vi "Construct Boolean Text Binding.vi"(7 "Format String":string, 10 "Bool Refnum":refnum<vi>) -> (0 "error out":errorcluster, 3 "BooleanTextBinding":refnum<class "BooleanTextBinding.lvclass">)   [LabVIEW 2020, in "BooleanTextBinding.lvclass"]
doc: "构造布尔文本绑定"
uses:
  BooleanTextBinding.lvclass
  BooleanTextBinding.lvclass/BooleanTextBinding.ctl
  <vilib>/Utility/error.llb/Error Cluster From Error Code.vi
  <vilib>/ErrorRing/Error Ring.xnode
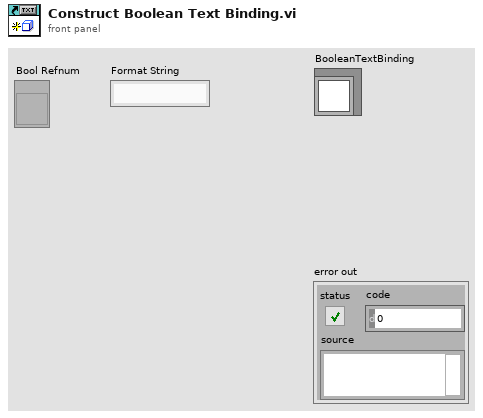
[diagram p1: front panel]
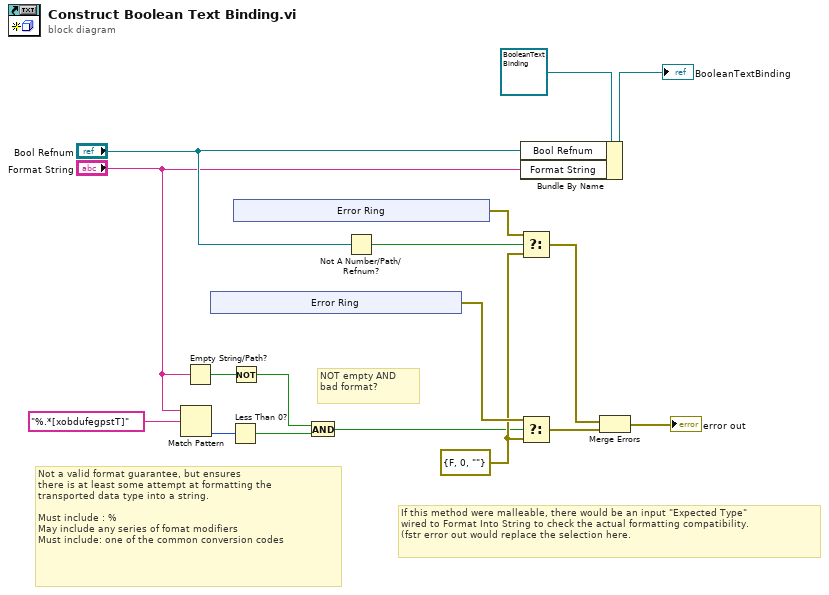
[diagram p0: block diagram]
diagram:
  w6 = errorcluster {"status"=FALSE, "code"=0, "source"=""} ("error constant")
  # "NOT empty AND\nbad format?"
  # "If this method were malleable, there would be an input \"Expected Type\"\nwired to Format Into String to check the actual formatting compatibility.\n(fstr error out would replace the selection here."
  # "Not a valid format guarantee, but ensures\nthere is at least some attempt at formatting the\ntransported data type into a string.\n\nMust include : %\nMay include any series of fomat modifiers\nMust include: one of the common conversion codes"
  n1 = Match Pattern(string="Format String", regular expression="%.*[xobdufegpstT]") -> (offset past match=w11:i32)  [unwired: 1 in, 3 out]
  n2 = Empty String/Path?(string/path="Format String") -> (empty?=w5:bool)
  n3 = xnode "Error Ring"() -> ("error out"=w10:errorcluster)
  n4 = Less Than 0?(x=w11) -> (x < 0?=w2:bool)
  n5 = Not(x=w5) -> (.not. x?=w4:bool)
  n6 = xnode "Error Ring"() -> ("error out"=w15:errorcluster)
  n7 = And(x=w4, y=w2) -> (x .and. y?=w1:bool)
  n8 = Not A Number/Path/Refnum?(number/path/refnum="Bool Refnum") -> (NaN/Path/Refnum?=w13:bool)
  n9 = Bundle By Name(cluster=refnum<class "BooleanTextBinding.lvclass"> refnum ("BooleanTextBinding"), "Bool Refnum"="Bool Refnum", "Format String"="Format String") -> (→"BooleanTextBinding":refnum<class "BooleanTextBinding.lvclass">)
  n10 = Select(t=w15, s=w13, f=w6) -> (s? t:f=w8:errorcluster)
  n11 = Select(t=w10, s=w1, f=w6) -> (s? t:f=w9:errorcluster)
  n12 = Merge Errors(w8, w9) -> (→"error out":errorcluster)
